vi "Read Binary Config.vi"(4 "Class Name is Included":bool, 6 "byte order (0:big-endian, network order)":T1(ring), 8 "error in (no error)":errorcluster, 10 "Binary":string, 11 "Const_DBL in":refnum<class "Const_DBL.lvclass">) -> (0 "error out":errorcluster, 2 "Remaining":string, 3 "Const_DBL out":refnum<class "Const_DBL.lvclass">)   [LabVIEW 2021, in "Const_DBL.lvclass"]
uses:
  Const_DBL.lvclass
  Const_DBL.lvclass/Const_DBL.ctl
  Abs_Types/Double Float/Abs_Double Float.lvclass
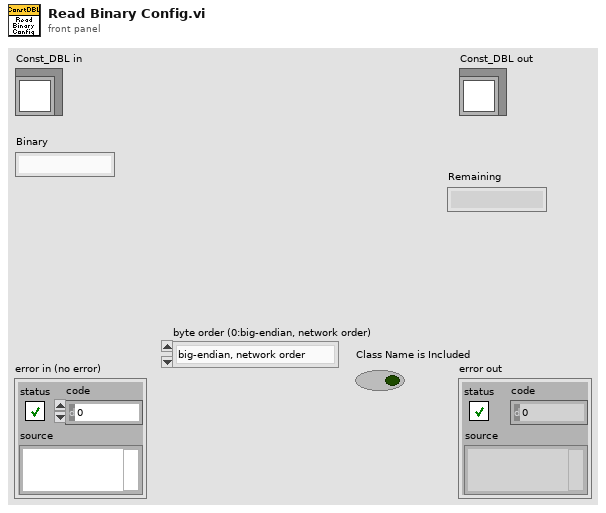
[diagram p1: front panel]
types:
  T1 = enum16{"big-endian, network order", "native, host order", "little-endian"}
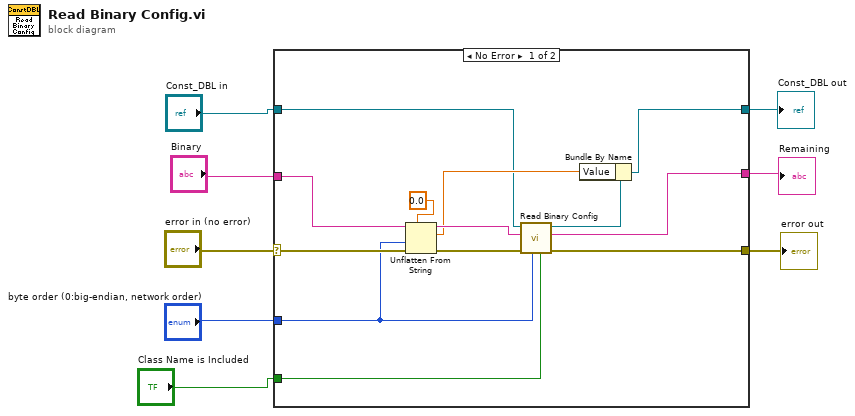
[diagram p0: block diagram]
diagram:
  n1 = case shown="No Error" "error in (no error)" {
    selector: "error in (no error)" -> [w19 w23]
    tunnel: [w14 w23] -> w3
    tunnel: [w11 w24] -> w1
    tunnel: "byte order (0:big-endian, network order)" -> [w16 _]
    tunnel: "Const_DBL in" -> [w13 w24]
    tunnel: "Binary" -> [w21 w22]
    tunnel: "Class Name is Included" -> [w10 _]
    tunnel: [w9 w22] -> w2
    frame No Error {
      n2 = Unflatten From String(type=0.0, binary string=w21, byte order (0:big-endian, network order)=w16, error in (no error)=w19) -> (rest of the binary string=w20:string, value=w17:dbl, error out=w18:errorcluster)  [unwired: 1 in]
      n3 = call-parent "Read Binary Config.vi"("Class Name is Included"=w10, "byte order (0:big-endian, network order)"=w16, "error in (no error)"=w18, "Binary"=w20, "Abs_Type in"=w13) -> ("error out"=w14:errorcluster, "Remaining"=w9:string, "Abs_Type out"=w12:refnum<class "Const_DBL.lvclass">)  [unwired: 4 in]
      n4 = Bundle By Name(cluster=w12, "Value"=w17) -> (w11:refnum<class "Const_DBL.lvclass">)
    }
    frame Error {
    }
  }
  "error out" <- w3
  "Const_DBL out" <- w1
  "Remaining" <- w2
